vi "Panel Destroy.vi"(8 "error in (no error)":errorcluster, 11 "Panel Control_Ref in":refnum<class "Panel Controller.lvclass">) -> (0 "error out":errorcluster, 3 "Panel Control_Ref out":refnum<class "Panel Controller.lvclass">)   [LabVIEW 2015, in "Panel Controller.lvclass"]
uses:
  Panel Controller.lvclass
  Panel GUI Manager/Panel GUI Manager.lvclass
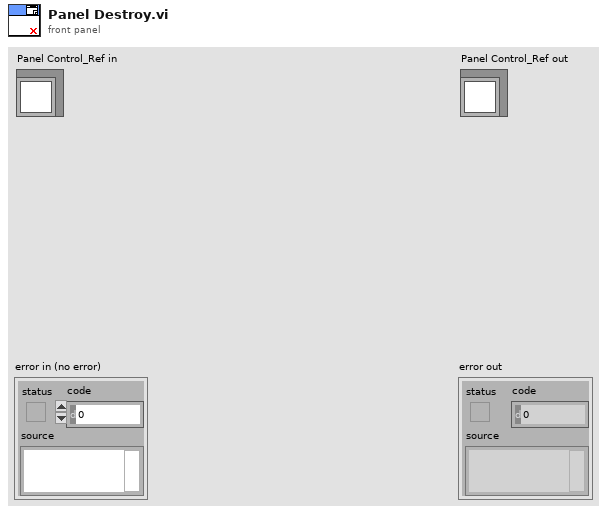
[diagram p1: front panel]
types:
  T1 = typedef "Panel Controller.lvclass/ObjectAttributes.ctl" = cluster{"Sub Panel Ref":refnum<vi>, "Panel_Q":refnum<queue>, "VI Running Refnum":refnum<vi>, "Brower Controller_Q":refnum<class "Message Enqueuer.lvclass">, "GUI Control Builder Director.lvclass":refnum<class "GUI Control Builder Director.lvclass">, "Panel GUI Manager.lvclass":refnum<class "Panel GUI Manager.lvclass">}
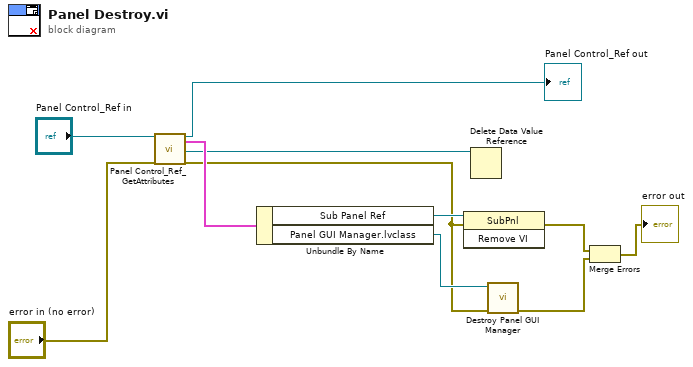
[diagram p0: block diagram]
diagram:
  n1 = call "Panel Control_Ref_GetAttributes.vi"("reference in"="Panel Control_Ref in", "error in (no error)"="error in (no error)") -> ("reference out"=→"Panel Control_Ref out":refnum<class "Panel Controller.lvclass">, "Data"=w9:T1, "DataRef"=w8:refnum<data-value>, "error out"=w4:errorcluster)  [unwired: 14 in]
  n2 = Unbundle By Name(w9) -> ("Sub Panel Ref"=w6:refnum<vi>, "Panel GUI Manager.lvclass"=w5:refnum<class "Panel GUI Manager.lvclass">)
  n3 = invoke class="SubPnl" method="Remove VI"(reference=w6, error in=w4) -> (error out=w3:errorcluster)  [unwired: 1 in, 2 out]
  n4 = Delete Data Value Reference(data value reference=w8) -> ()  [unwired: 1 in, 2 out]
  n5 = call "Destroy Panel GUI Manager.vi"("error in (no error)"=w4, "Panel GUI Manager in"=w5) -> ("error out"=w2:errorcluster)  [unwired: 8 in, 1 out]
  n6 = Merge Errors(w3, w2) -> (→"error out":errorcluster)
